vi "ClientV2.vi"() -> ()   [LabVIEW 2021]
panel:
  in  "Ultra CHARGE":dbl(knob) scale=0.0..100.0
  in  "Ultraman Chest Powa":bool
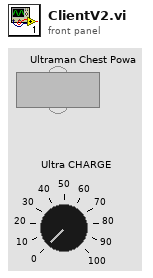
[diagram p1: front panel]
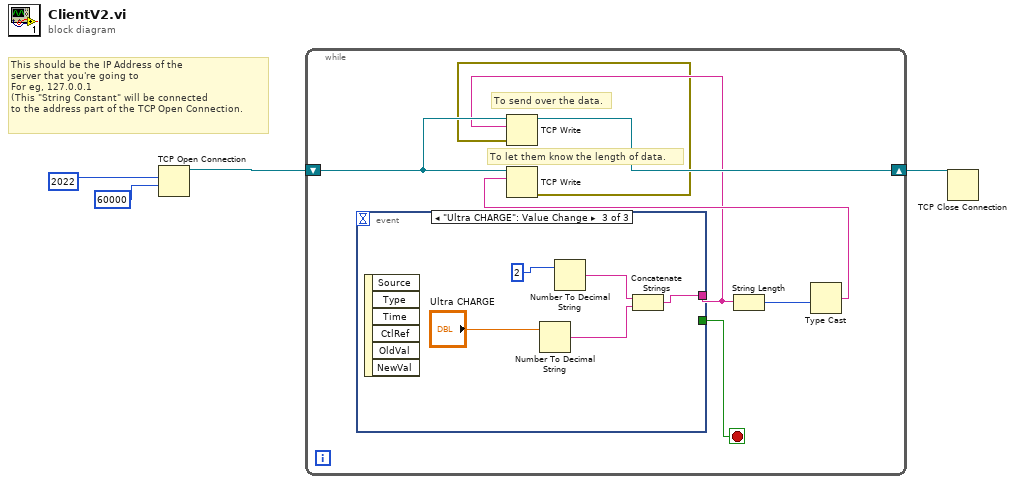
[diagram p0: block diagram]
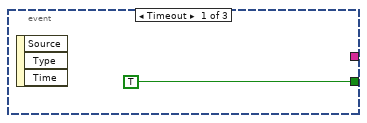
[diagram p2: hidden frame]
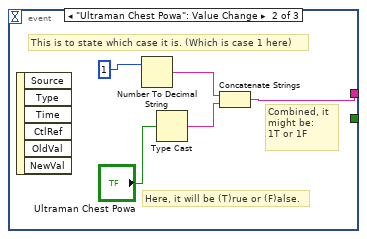
[diagram p3: hidden frame]
diagram:
  # "This should be the IP Address of the\nserver that you're going to\nFor eg, 127.0.0.1 \n(This \"String Constant\" will be connected\nto the address part of the TCP Open Connection."
  n1 = TCP Open Connection(remote port or service name=2022, timeout ms (60000)=60000) -> (connection ID=w2:refnum<k5>)  [unwired: 3 in, 1 out]
  n2 = while {
    shift-right: [w10] -> w1
    shift-left: w2 -> [w11]
    stop <- w9 stop-if-true
    # "To send over the data."
    # "To let them know the length of data."
    n3 = event shown="[2] \"Ultra CHARGE\": Value Change" {
      selector: _ -> [_ _ _]
      dyn-events: _ -> [_ _ _]
      timeout: _ -> [_ _ _]
      tunnel: [TRUE _ _] -> w9
      tunnel: [_ w13 w18] -> w6
      event Timeout {
        n4 = event-data() -> ()  [unwired: 1 in, 3 out]
      }
      event "Ultraman Chest Powa": Value Change {
        # "Combined, it\nmight be:\n1T or 1F"
        # "Here, it will be (T)rue or (F)alse."
        # "This is to state which case it is. (Which is case 1 here)"
        n5 = event-data() -> ()  [unwired: 1 in, 6 out]
        n6 = Number To Decimal String(number=1) -> (decimal integer string=w15:string)  [unwired: 1 in]
        n7 = Type Cast(x="Ultraman Chest Powa") -> (*(type *) &x=w14:string)  [unwired: 1 in]
        n8 = Concatenate Strings(w15, w14) -> (w13:string)
      }
      event "Ultra CHARGE": Value Change {
        n9 = event-data() -> ()  [unwired: 1 in, 6 out]
        n10 = Number To Decimal String(number="Ultra CHARGE") -> (decimal integer string=w19:string)  [unwired: 1 in]
        n11 = Number To Decimal String(number=2) -> (decimal integer string=w21:string)  [unwired: 1 in]
        n12 = Concatenate Strings(w21, w19) -> (w18:string)
      }
    }
    n13 = String Length(string=w6) -> (length=w8:i32)
    n14 = Type Cast(x=w8) -> (*(type *) &x=w7:string)  [unwired: 1 in]
    n15 = TCP Write(connection ID=w11, data in=w7) -> (error out=w5:errorcluster)  [unwired: 2 in, 2 out]
    n16 = TCP Write(connection ID=w11, data in=w6, error in (no error)=w5) -> (connection ID out=w10:refnum<k5>)  [unwired: 1 in, 2 out]
  }
  n17 = TCP Close Connection(connection ID=w1) -> ()  [unwired: 2 in, 2 out]
